vi "dfd_DFXP SymAccAdd (vector).vi"(10 "Values in":T1, 11 "Acc":T2={"value"=0, "wl"=0, "iwl"=0, "Signed"=TRUE} {"value" format="%.0x"}) -> (3 "Value out":T2={"value"=0, "wl"=0, "iwl"=0, "Signed"=TRUE} {"value" format="%.0x"})   [LabVIEW 2017, in "NI_DigFilter_FXP.lvlib"]
uses:
  <vilib>/addons/Digital Filter Design/NI_DigFilter_FXP.lvlib
  <vilib>/addons/Digital Filter Design/_Objects.llb/dfd_DFXP Data Type (scaler).ctl
  <vilib>/addons/Digital Filter Design/_Objects.llb/dfd_DFXP Data Type (vector).ctl
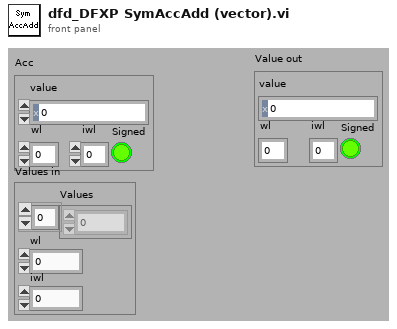
[diagram p1: front panel]
types:
  T1 = typedef "dfd_DFXP Data Type (vector).ctl" = cluster{"Values":i64[], "wl":i16, "iwl":i16}
  T2 = typedef "dfd_DFXP Data Type (scaler).ctl" = cluster{"value":i64, "wl":i16, "iwl":i16, "Signed":bool}
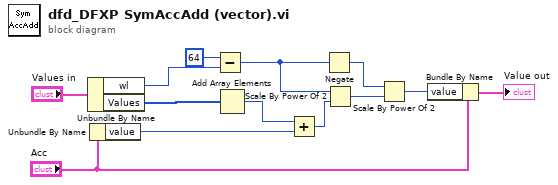
[diagram p0: block diagram]
diagram:
  n1 = Unbundle By Name("Values in") -> ("wl"=w1:i16, "Values"=w11:i64[])
  n2 = Unbundle By Name("Acc") -> ("value"=w5:i64)
  n3 = Subtract(x=i16 64, y=w1) -> (x-y=w8:i16)
  n4 = Add Array Elements(numeric array=w11) -> (sum=w4:i64)
  n5 = Add(x=w4, y=w5) -> (x+y=w3:i64)
  n6 = Negate(x=w8) -> (-x=w7:i16)
  n7 = Scale By Power Of 2(n=w8, x=w3) -> (x*2^n=w9:i64)
  n8 = Scale By Power Of 2(n=w7, x=w9) -> (x*2^n=w2:i64)
  n9 = Bundle By Name(cluster="Acc", "value"=w2) -> (→"Value out":T2)
